vi "SLL DE Split Virtual Channels based on Device v1.vi"(8 "error in (no error)":errorcluster, 11 "GlobalChans":refnum<k21>[](array[refnum])) -> (0 "error out":errorcluster, 2 "Channel Array":cluster{"Device Channel List":string[]}[](array[cluster]), 3 "Devices Names":string[](array[string]))   [LabVIEW 2013]
doc: "This VI will split channels based on its Device ID.\nFor each device, this VI will list channels in 1D array. and then Build 2D Array for all device.\n\nCreated by Yogesh Redemptor, \nCopyright © 2008, Soliton Technologies.\nAll rights reserved."
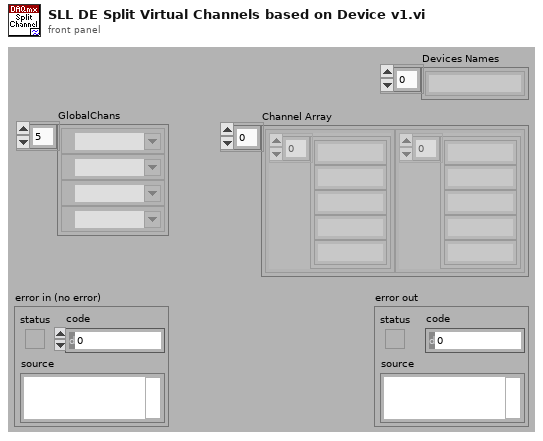
[diagram p1: front panel]
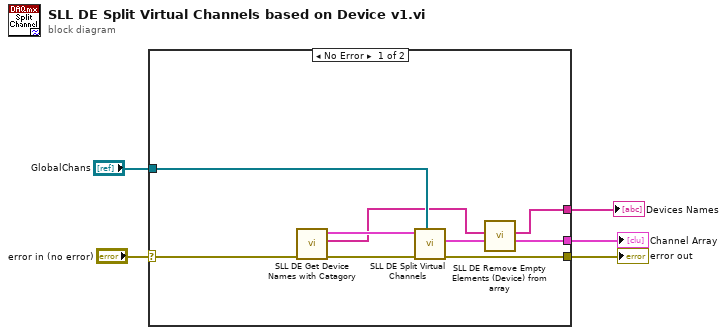
[diagram p0: block diagram]
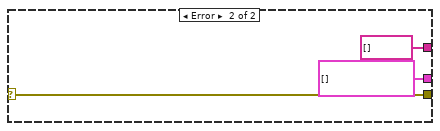
[diagram p2: hidden frame]
diagram:
  n1 = case shown="No Error" "error in (no error)" {
    selector: "error in (no error)" -> [w10 w17]
    tunnel: [w7 cluster{"Device Channel List":string[]}[] [] ("Channel Array")] -> w5
    tunnel: [w14 w17] -> w4
    tunnel: [w6 string[] [] ("Devices Names")] -> w3
    tunnel: "GlobalChans" -> [w11 _]
    frame No Error {
      n2 = call "SLL DE Get Device Names with Catagory.vi"("error in (no error)"=w10) -> ("error out"=w13:errorcluster, "Devices Names"=w9:string[], "All Device Names (Chassis & Module)"=w12:cluster{"New element":tag[]}[])  [unwired: 8 in]
      n3 = call "SLL DE Split Virtual Channels.vi"("GlobalChans"=w11, "error in (no error)"=w13, "All Device Names (Chassis & Module)"=w12) -> ("error out"=w14:errorcluster, "Channel Array"=w8:cluster{"Device Channel List":string[]}[])  [unwired: 6 in, 1 out]
      n4 = call "SLL DE Remove Empty Elements (Device) from array.vi"("Channel ArrayIn"=w8, "Devices Names In"=w9) -> ("Channel Array Out"=w7:cluster{"Device Channel List":string[]}[], "Devices Names"=w6:string[])  [unwired: 8 in]
    }
    frame Error {
    }
  }
  "Channel Array" <- w5
  "Devices Names" <- w3
  "error out" <- w4
